vi "Set Read Timeout.vi"(8 "error in (no error)":errorcluster, 10 "read operation timeout":i32=5000, 11 "Modbus master in":refnum<class "Modbus Master.lvclass">) -> (0 "error out":errorcluster, 3 "Modbus master out":refnum<class "Modbus Master.lvclass">)   [LabVIEW 2018, in "Modbus Master.lvclass"]
doc: "<B>Read Timeout</B> specifies the read operation timeout. You can use a Modbus master instance to perform read operations on a Modbus slave with the specified timeout."
uses:
  Modbus Master.lvclass
  C:/Program Files (x86)/National Instruments/LabVIEW 2018/vi.lib/Modbus/subvis/Modbus API/Modbus API.lvclass
  Modbus API.lvclass/Modbus API.ctl
  Transmission Data Unit.lvclass/Transmission Data Unit.ctl
  Transmission Data Unit.lvclass
  Modbus API.lvclass
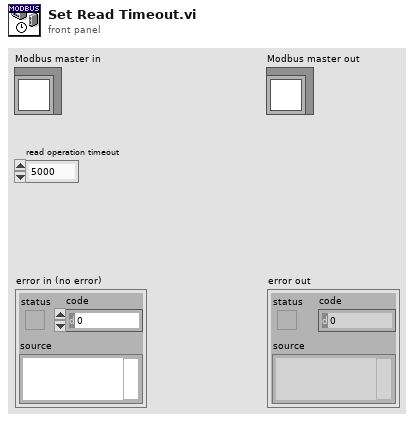
[diagram p1: front panel]
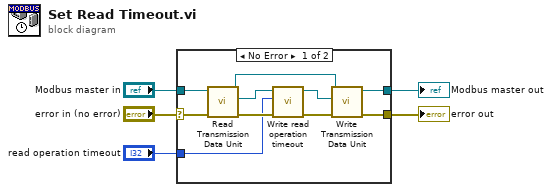
[diagram p0: block diagram]
diagram:
  n1 = case shown="No Error" "error in (no error)" {
    selector: "error in (no error)" -> [w6 w16]
    tunnel: "read operation timeout" -> [w10 _]
    tunnel: [w9 w17] -> w4
    tunnel: "Modbus master in" -> [w8 w17]
    tunnel: [w7 w16] -> w2
    frame No Error {
      n2 = call "Read Transmission Data Unit.vi"("error in (no error)"=w6, "Modbus instance in"=w8) -> ("error out"=w11:errorcluster, "transmission data unit"=w14:refnum<class "Transmission Data Unit.lvclass">, "Modbus instance out"=w15:refnum<class "Modbus Master.lvclass">)  [unwired: 7 in]
      n3 = call "Write read operation timeout.vi"("error in (no error)"=w11, "read operation timeout"=w10, "transmission data unit in"=w14) -> ("error out"=w12:errorcluster, "transmission data unit out"=w13:refnum<class "Transmission Data Unit.lvclass">)  [unwired: 7 in]
      n4 = call "Write Transmission Data Unit.vi"("error in (no error)"=w12, "transmission data unit"=w13, "Modbus instance in"=w15) -> ("error out"=w7:errorcluster, "Modbus instance out"=w9:refnum<class "Modbus Master.lvclass">)  [unwired: 7 in]
    }
    frame Error {
    }
  }
  "error out" <- w2
  "Modbus master out" <- w4
